vi "Update Enable.vi"(8 "error in (no error)":errorcluster, 10 "Station Status":map{string, bool}(c390), 11 "Update OPC Server in":refnum<class "OPC Server.lvclass">) -> (0 "error out":errorcluster, 3 "Update OPC Server out":refnum<class "OPC Server.lvclass">)   [LabVIEW 2021, in "OPC Server.lvlib" / "OPC Server.lvclass"]
uses:
  OPC Server.lvclass
  OPC Server.lvclass/OPC Server.ctl
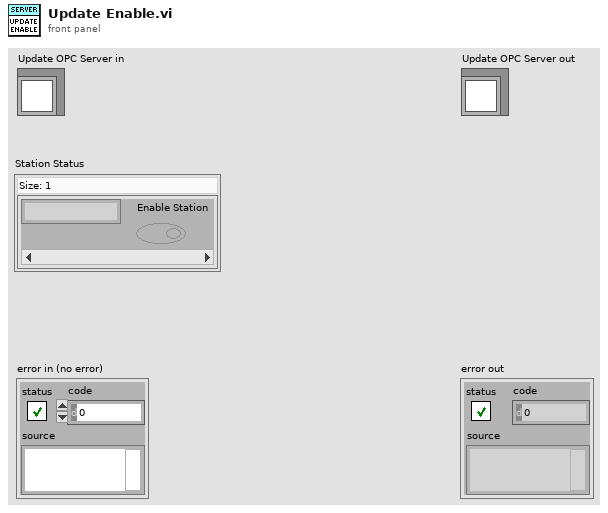
[diagram p1: front panel]
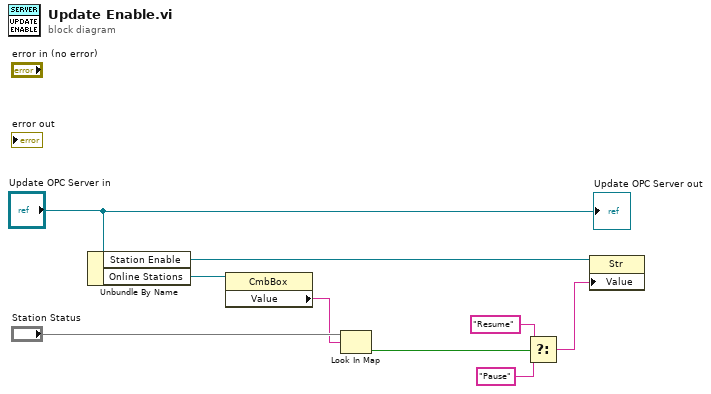
[diagram p0: block diagram]
diagram:
  n1 = Unbundle By Name("Update OPC Server in") -> ("Station Enable"=w8:refnum<vi>, "Online Stations"=w6:refnum<vi>)
  n2 = property class="CmbBox"(reference=w6) -> ("Value"=w5:string)  [unwired: 1 in, 2 out]
  n3 = Look In Map(map="Station Status", key=w5) -> (value=w1:bool)  [unwired: 1 in, 1 out]
  n4 = Select(t="Resume" ("Value"), s=w1, f="Pause" ("Value")) -> (s? t:f=w2:string)
  n5 = property class="Str"(reference=w8, "Value"=w2) -> ()  [unwired: 1 in, 2 out]
  "Update OPC Server out" <- "Update OPC Server in"
